vi "Add Monitoring Channels.vi"(8 "Error In":errorcluster, 11 "Port Section Item Ref in":T1 format="%.0x") -> (0 "Error Out":errorcluster, 3 "Port Section Item Ref Out":T1 format="%.0x")   [LabVIEW 2018, in "NI-XNET Monitor System Explorer.lvlib"]
uses:
  NI-XNET Monitor System Explorer.lvlib
  <vilib>/NI Veristand/Custom Device API/Custom Device Item Ref.ctl
  <vilib>/NI Veristand/Custom Device API/Custom Device Channel.ctl
  <vilib>/NI Veristand/Custom Device API/Custom Device Channel Type.ctl
  Shared/Constants.vi
  <vilib>/NI Veristand/Custom Device API/Custom Device API.lvlib
  Shared/NI-XNET Monitor Shared.lvlib
  <vilib>/xnet/xnet.llb/XNET CAN Last Err.ctl
  <vilib>/xnet/xnet.llb/XNET CAN Comm State.ctl
  <vilib>/xnet/xnet.llb/XNET FlexRay POC State.ctl
  <vilib>/xnet/xnet.llb/XNET LIN Last Err.ctl
  <vilib>/xnet/xnet.llb/XNET LIN Comm State.ctl
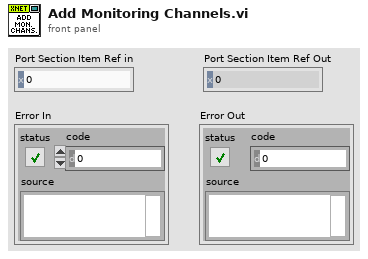
[diagram p1: front panel]
types:
  T1 = typedef "Custom Device API.lvlib/Custom Device Item Ref.ctl" = u64
  T2 = typedef "Custom Device API.lvlib/Custom Device Channel.ctl" = cluster{"Type":T3, "Units":string, "Default Value":dbl, "Faultable":bool, "Scalable":bool}
  T3 = typedef "Custom Device API.lvlib/Custom Device Channel Type.ctl" = enum16{"Input", "Output"}
  T4 = typedef "Custom Device API.lvlib/Custom Device Item Info.ctl" = cluster{"Name":string, "Is Channel":bool, "GUID":string, "Is Waveform":bool}
  T5 = typedef "XNET CAN Comm State.ctl" = u8
  T6 = typedef "XNET CAN Last Err.ctl" = u8
  T7 = cluster{"fault code":i32, "communication state":T5, "last error":T6, "receive error counter":u8, "transmit error counter":u8}
  T8 = typedef "XNET FlexRay POC State.ctl" = u8
  T9 = cluster{"fault code":i32, "FlexRay POC state":T8, "clock correction failed":u8, "passive to active count":u8}
  T10 = typedef "XNET LIN Comm State.ctl" = u8
  T11 = typedef "XNET LIN Last Err.ctl" = u8
  T12 = cluster{"fault code":i32, "communication state":T10, "last error":T11, "last error received":u8, "last error expected":u8, "last error identifier":u8, "schedule index":u8}
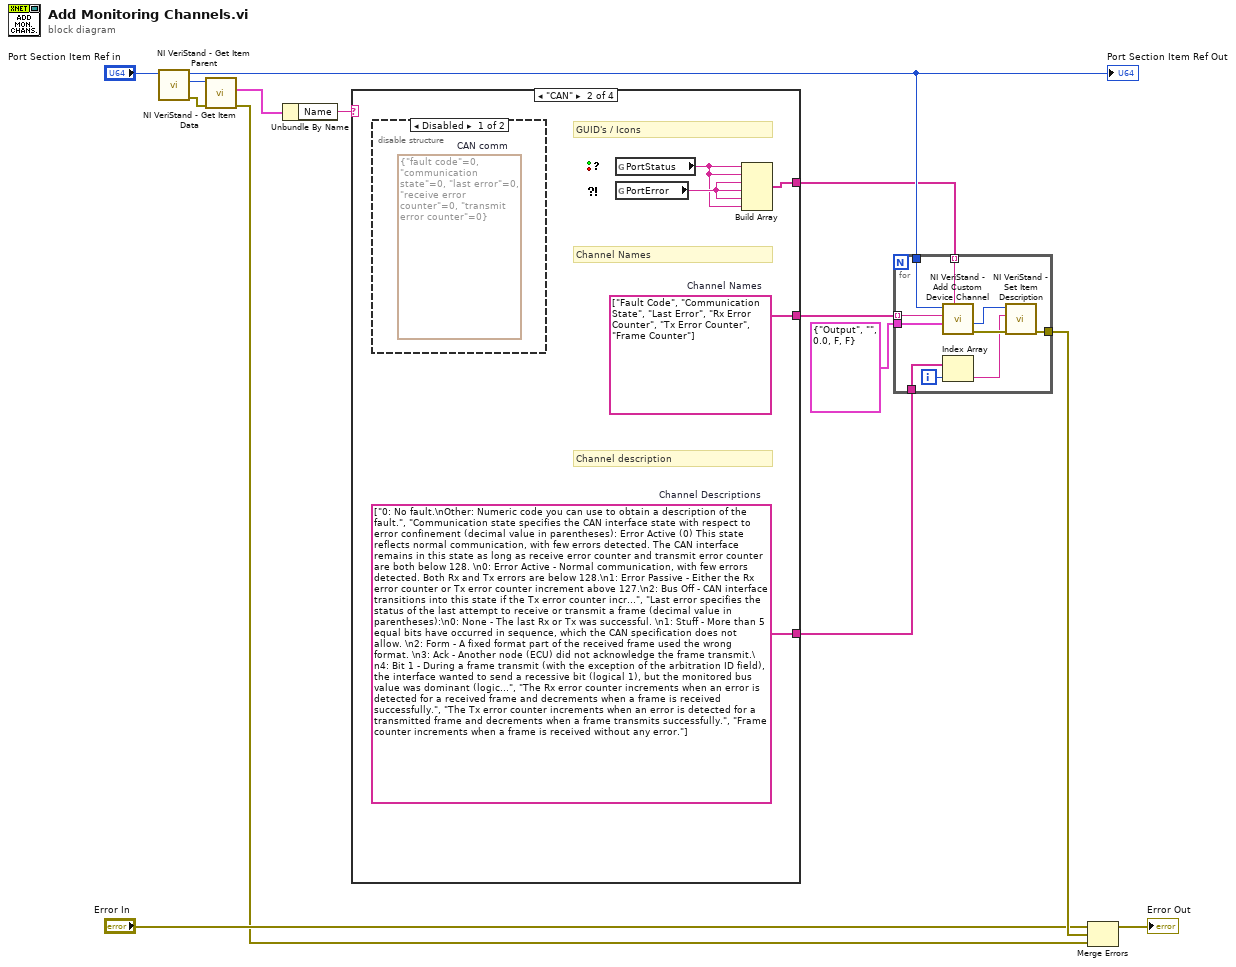
[diagram p0: block diagram]
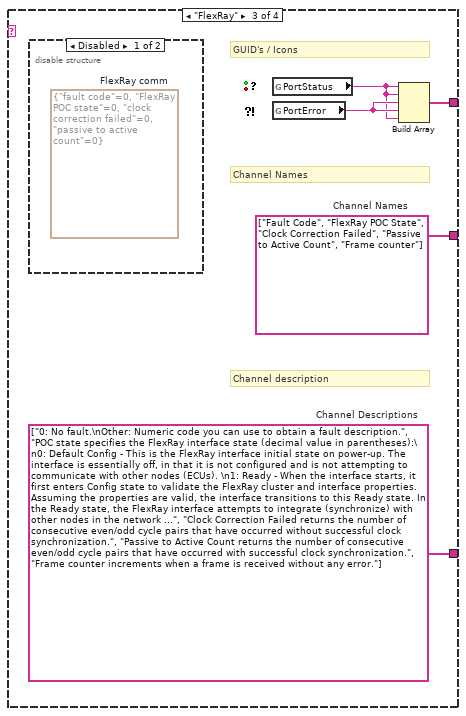
[diagram p4: hidden frame]
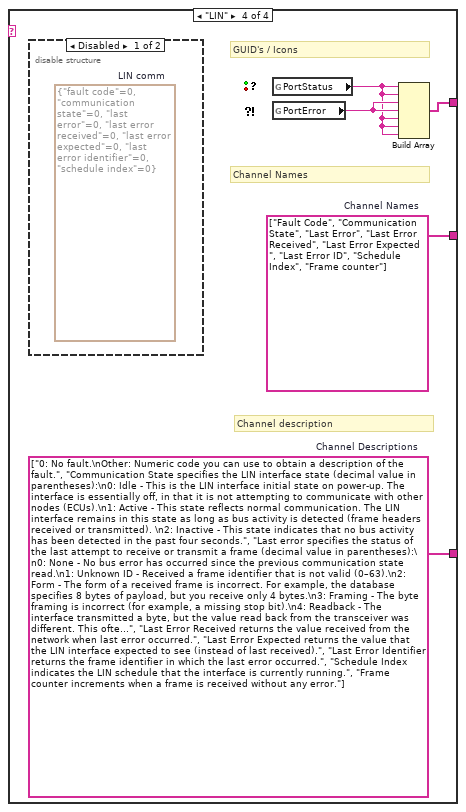
[diagram p6: hidden frame]
diagram:
  n1 = call <vilib>:"NI VeriStand - Get Item Parent.vi"("Item Ref in"="Port Section Item Ref in") -> ("error out"=w11:errorcluster, "Parent Ref"=w12:T1, "Item Ref out"=w13:T1)  [unwired: 7 in, 1 out]
  "Port Section Item Ref Out" <- w13
  n2 = call <vilib>:"NI VeriStand - Get Item Data.vi"("error in (no error)"=w11, "Item Ref in"=w12) -> ("error out"=w2:errorcluster, "Item Info"=w10:T4)  [unwired: 6 in, 2 out]
  n3 = Unbundle By Name(w10) -> ("Name"=w9:string)
  n4 = case shown="\"CAN\"" w9 {
    tunnel: [_ w18 w24 w28] -> w7
    tunnel: [_ w17 w23 w27] -> w6
    tunnel: [_ w16 w22 w26] -> w5
    frame Default {
      # "Should never happen"
    }
    frame "CAN" {
      w16 = string[] ["0: No fault.\nOther: Numeric code you can use to obtain a description of the fault.", "Communication state specifies the CAN interface state with respect to error confinement (decimal value in parentheses): Error Active (0) This state reflects normal communication, with few errors detected. The CAN interface remains in this state as long as receive error counter and transmit error counter are both below 128. \n0: Error Active - Normal communication, with few errors detected. Both Rx and Tx errors are below 128.\n1: Error Passive - Either the Rx error counter or Tx error counter increment above 127.\n2: Bus Off - CAN interface transitions into this state if the Tx error counter increments above 255.\n3: Init - CAN interface initial state on power-up.", "Last error specifies the status of the last attempt to receive or transmit a frame (decimal value in parentheses):\n0: None - The last Rx or Tx was successful. \n1: Stuff - More than 5 equal bits have occurred in sequence, which the CAN specification does not allow. \n2: Form - A fixed format part of the received frame used the wrong format. \n3: Ack - Another node (ECU) did not acknowledge the frame transmit.\n4: Bit 1 - During a frame transmit (with the exception of the arbitration ID field), the interface wanted to send a recessive bit (logical 1), but the monitored bus value was dominant (logical 0). \n5: Bit 0 - During a frame transmit (with the exception of the arbitration ID field), the interface wanted to send a dominant bit (logical 0), but the monitored bus value was recessive (logical 1). \n6: CRC - The CRC contained within a received frame does not match the CRC calculated for the incoming bits.", "The Rx error counter increments when an error is detected for a received frame and decrements when a frame is received successfully.", "The Tx error counter increments when an error is detected for a transmitted frame and decrements when a frame transmits successfully.", "Frame counter increments when a frame is received without any error."]  # Channel Descriptions
      w18 = string[] ["Fault Code", "Communication State", "Last Error", "Rx Error Counter", "Tx Error Counter", "Frame Counter"]  # Channel Names
      # "Channel description"
      # "Channel Names"
      # "GUID's / Icons"
      n5 = disable-structure shown="Disabled" {
        frame Disabled {
          (unwired) T7 {"fault code"=0, "communication state"=0, "last error"=0, "receive error counter"=0, "transmit error counter"=0}  # CAN comm
        }
        frame Enabled {
        }
      }
      n6 = global read "Constants.vi" "PortStatus"() -> (w15:string)
      n7 = global read "Constants.vi" "PortError"() -> (w19:string)
      n8 = Build Array(w15, w15, w19, w19, w19, w15) -> (w17:string[])
    }
    frame "FlexRay" {
      w22 = string[] ["0: No fault.\nOther: Numeric code you can use to obtain a fault description.", "POC state specifies the FlexRay interface state (decimal value in parentheses):\n0: Default Config - This is the FlexRay interface initial state on power-up. The interface is essentially off, in that it is not configured and is not attempting to communicate with other nodes (ECUs). \n1: Ready - When the interface starts, it first enters Config state to validate the FlexRay cluster and interface properties. Assuming the properties are valid, the interface transitions to this Ready state. In the Ready state, the FlexRay interface attempts to integrate (synchronize) with other nodes in the network cluster. This integration process can take several FlexRay cycles, up to 200 ms. If the integration succeeds, the interface transitions to Normal Active.\n\n2: Normal Active - This is the normal operation state. The NI-XNET interface is adequately synchronized to the cluster to allow continued frame transmission without disrupting the transmissions of other nodes (ECUs). If synchronization problems occur, the interface can transition from this state to Normal Passive.\n3: Normal Passive - Frame reception is allowed, but frame transmission is disabled due to degraded synchronization with the cluster remainder. If synchronization improves, the interface can transition to Normal Active. If synchronization continues to degrade, the interface transitions to Halt.\n4: Halt - Communication halted due to synchronization problems.\n15: Config - This state is transitional when configuration is valid. If you detect this state after starting the interface, it typically indicates a problem with the configuration. Check the fault? output for a fault. If no fault is returned, check your FlexRay cluster and interface properties. You can check the validity of these properties using the NI-XNET Database Editor, which displays invalid configuration properties.", "Clock Correction Failed returns the number of consecutive even/odd cycle pairs that have occurred without successful clock synchronization.", "Passive to Active Count returns the number of consecutive even/odd cycle pairs that have occurred with successful clock synchronization.", "Frame counter increments when a frame is received without any error."]  # Channel Descriptions
      w24 = string[] ["Fault Code", "FlexRay POC State", "Clock Correction Failed", "Passive to Active Count", "Frame counter"]  # Channel Names
      # "Channel description"
      # "Channel Names"
      # "GUID's / Icons"
      n9 = disable-structure shown="Disabled" {
        frame Disabled {
          (unwired) T9 {"fault code"=0, "FlexRay POC state"=0, "clock correction failed"=0, "passive to active count"=0}  # FlexRay comm
        }
        frame Enabled {
        }
      }
      n10 = global read "Constants.vi" "PortStatus"() -> (w20:string)
      n11 = global read "Constants.vi" "PortError"() -> (w21:string)
      n12 = Build Array(w20, w20, w21, w21, w20) -> (w23:string[])
    }
    frame "LIN" {
      w26 = string[] ["0: No fault.\nOther: Numeric code you can use to obtain a description of the fault.", "Communication State specifies the LIN interface state (decimal value in parentheses):\n0: Idle - This is the LIN interface initial state on power-up. The interface is essentially off, in that it is not attempting to communicate with other nodes (ECUs).\n1: Active - This state reflects normal communication. The LIN interface remains in this state as long as bus activity is detected (frame headers received or transmitted). \n2: Inactive - This state indicates that no bus activity has been detected in the past four seconds.", "Last error specifies the status of the last attempt to receive or transmit a frame (decimal value in parentheses):\n0: None - No bus error has occurred since the previous communication state read.\n1: Unknown ID - Received a frame identifier that is not valid (0–63).\n2: Form - The form of a received frame is incorrect. For example, the database specifies 8 bytes of payload, but you receive only 4 bytes.\n3: Framing - The byte framing is incorrect (for example, a missing stop bit).\n4: Readback - The interface transmitted a byte, but the value read back from the transceiver was different. This often is caused by a cabling problem, such as noise.\n5: Timeout - Receiving the frame took longer than the LIN-specified timeout.\n6: Checksum - The received checksum was different than the expected checksum.", "Last Error Received returns the value received from the network when last error occurred.", "Last Error Expected returns the value that the LIN interface expected to see (instead of last received).", "Last Error Identifier returns the frame identifier in which the last error occurred.", "Schedule Index indicates the LIN schedule that the interface is currently running.", "Frame counter increments when a frame is received without any error."]  # Channel Descriptions
      w28 = string[] ["Fault Code", "Communication State", "Last Error", "Last Error Received", "Last Error Expected ", "Last Error ID", "Schedule Index", "Frame counter"]  # Channel Names
      # "Channel description"
      # "Channel Names"
      # "GUID's / Icons"
      n13 = disable-structure shown="Disabled" {
        frame Disabled {
          (unwired) T12 {"fault code"=0, "communication state"=0, "last error"=0, "last error received"=0, "last error expected"=0, "last error identifier"=0, "schedule index"=0}  # LIN comm
        }
        frame Enabled {
        }
      }
      n14 = global read "Constants.vi" "PortStatus"() -> (w25:string)
      n15 = global read "Constants.vi" "PortError"() -> (w29:string)
      n16 = Build Array(w25, w25, w29, w29, w25, w25, w25) -> (w27:string[])
    }
  }
  n17 = for {
    tunnel: w13 -> [w39]
    tunnel: [w36] -> w8
    tunnel: w7 -> [w35] mode=indexing
    tunnel: w6 -> [w34] mode=indexing
    tunnel: w5 -> [w31]
    tunnel: T2 {"Type"=enum."Output", "Units"="", "Default Value"=0.0, "Faultable"=FALSE, "Scalable"=FALSE} ("Channel") -> [w30]
    i -> [w32]
    n18 = call <vilib>:"NI VeriStand - Add Custom Device Channel.vi"("GUID (Default Channel)"=w34, "Channel"=w30, "Channel Name"=w35, "Parent Ref in"=w39) -> ("error out"=w37:errorcluster, "Channel Ref"=w38:T1)  [unwired: 4 in, 2 out]
    n19 = Index Array(array=w31, index=w32) -> (element=w33:string)
    n20 = call <vilib>:"NI VeriStand - Set Item Description.vi"("error in (no error)"=w37, "Description"=w33, "Item Ref in"=w38) -> ("error out"=w36:errorcluster)  [unwired: 6 in, 2 out]
  }
  n21 = Merge Errors("Error In", w8, w2) -> (→"Error Out":errorcluster)
